vi "MainCode.vi"() -> ()   [LabVIEW 2022 SP3]
uses:
  <vilib>/Instr/_visa.llb/VISA Configure Serial Port (Instr).vi
panel:
  out "Array":string[](array[string])
  in  "Test":bool
  in  "OK Button":bool
  out "read buffer":string="import sensor, image, time\r\n>>> \r\n>>> sensor.reset()\r\n>>> sensor.set_pixformat(sensor.RGB565)\r\nTrue\r\n>>> sensor.set_framesize(sensor.QVGA)  \r\nTrue\r\n>>> sensor.skip_frames(time = 2000)\r\n>>> img = sensor.snapshot()\r\n>>> \r\n>>> \r\n>>> \r\n>>> \r\n>>> "
  out "value":u32[](array[numeric])=[1869639017, 1931506802, 1869835877, 1763716210, 1701273965, 1769218092, 168650093, 540950078, 1044253197, 1702043710, 1919906670, 1936028206, 690517093, 1044253197, 1702043710, 1919906670, 1952805678, 2020175967, 1836216166, 1932031073, 1869835877, 1196568178, 892745026, 1409944873, 224753010, 1044266506, 1852142368, 779251571, 1601463667, 1835102822, 2053731173, 1702045797, 1919906670, 1196839214, 538978625, 1918110221, 168650101, 540950078, 1936614771, 1932423791, 1601202539, 1835102822, 1948808037, 543518057, 808591421, 220803120, 1044266506, 1735223584, 1931492640, 1869835877, 1853042290, 1752395873, 690517103, 1044253197, 168632382, 540950078, 1044253197, 168632382, 540950078, 1044253197] format="%.0x"
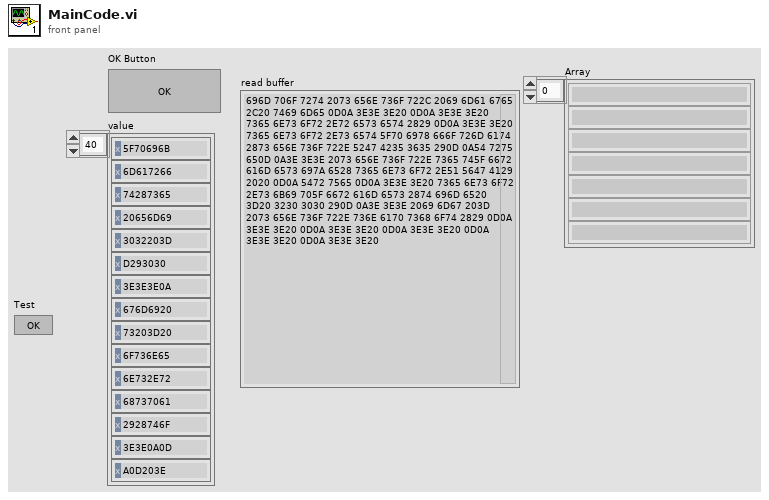
[diagram p1: front panel]
types:
  T1 = enum16{"big-endian, network order", "native, host order", "little-endian"}
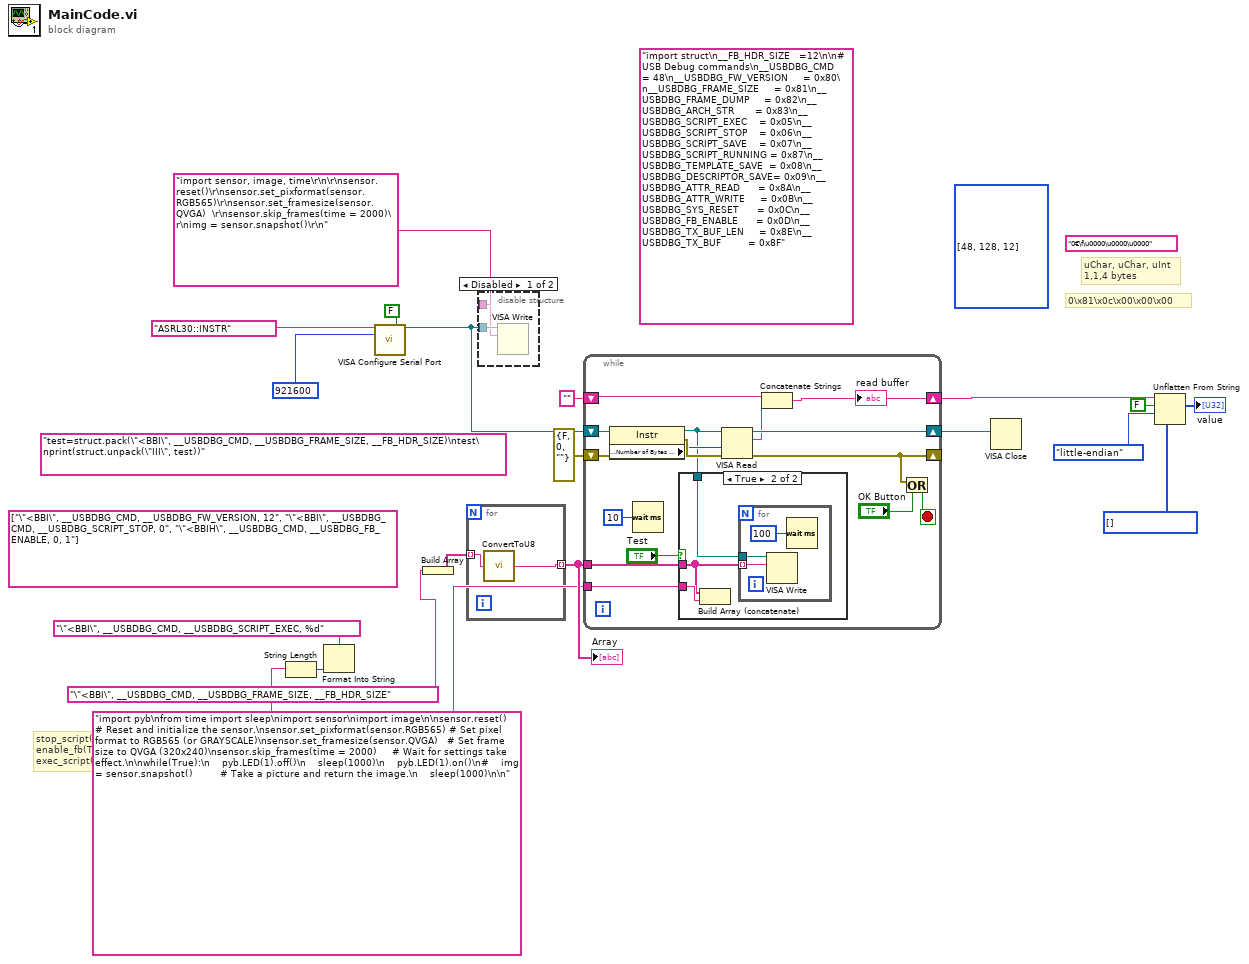
[diagram p0: block diagram]
diagram:
  w3 = "import pyb\nfrom time import sleep\nimport sensor\nimport image\n\nsensor.reset()                      # Reset and initialize the sensor.\nsensor.set_pixformat(sensor.RGB565) # Set pixel format to RGB565 (or GRAYSCALE)\nsensor.set_framesize(sensor.QVGA)   # Set frame size to QVGA (320x240)\nsensor.skip_frames(time = 2000)     # Wait for settings take effect.\n\nwhile(True):\n    pyb.LED(1).off()\n    sleep(1000)\n    pyb.LED(1).on()\n#    img = sensor.snapshot()         # Take a picture and return the image.\n    sleep(1000)\n\n" ("header buffer")
  (unwired) string[] ["\"<BBI\", __USBDBG_CMD, __USBDBG_FW_VERSION, 12", "\"<BBI\", __USBDBG_CMD, __USBDBG_SCRIPT_STOP, 0", "\"<BBIH\", __USBDBG_CMD, __USBDBG_FB_ENABLE, 0, 1"]
  (unwired) i32[] [48, 128, 12]
  (unwired) "0€\f\u0000\u0000\u0000" ("Last")
  (unwired) "test=struct.pack(\"<BBI\", __USBDBG_CMD, __USBDBG_FRAME_SIZE, __FB_HDR_SIZE)\ntest\nprint(struct.unpack(\"III\", test))" ("write buffer")
  (unwired) "import struct\n__FB_HDR_SIZE   =12\n\n# USB Debug commands\n__USBDBG_CMD            = 48\n__USBDBG_FW_VERSION     = 0x80\n__USBDBG_FRAME_SIZE     = 0x81\n__USBDBG_FRAME_DUMP     = 0x82\n__USBDBG_ARCH_STR       = 0x83\n__USBDBG_SCRIPT_EXEC    = 0x05\n__USBDBG_SCRIPT_STOP    = 0x06\n__USBDBG_SCRIPT_SAVE    = 0x07\n__USBDBG_SCRIPT_RUNNING = 0x87\n__USBDBG_TEMPLATE_SAVE  = 0x08\n__USBDBG_DESCRIPTOR_SAVE= 0x09\n__USBDBG_ATTR_READ      = 0x8A\n__USBDBG_ATTR_WRITE     = 0x0B\n__USBDBG_SYS_RESET      = 0x0C\n__USBDBG_FB_ENABLE      = 0x0D\n__USBDBG_TX_BUF_LEN     = 0x8E\n__USBDBG_TX_BUF         = 0x8F" ("write buffer")
  # "\"<BBI\", __USBDBG_CMD, __USBDBG_SCRIPT_EXEC, len(buf))"
  # "stop_script()\nenable_fb(True)\nexec_script(script)"
  # "uChar, uChar, uInt\n1,1,4 bytes"
  # "0\\x81\\x0c\\x00\\x00\\x00"
  n1 = String Length(string=w3) -> (length=w4:i32)
  n2 = Format Into String(format string="\"<BBI\", __USBDBG_CMD, __USBDBG_SCRIPT_EXEC, %d" ("write buffer"), w4) -> ()  [unwired: 2 in, 2 out]
  n3 = call-poly "VISA Configure Serial Port"("VISA resource name"="ASRL30::INSTR" ("Serial Address"), "Enable Termination\nChar (T)"=FALSE ("Enable Termination\nChar (T)"), "baud rate (9600)"=u32 921600 ("baud rate (115200)")) -> ("VISA resource name out"=w12:refnum<visa-resource-name>)  [unwired: 11 in, 1 out]
  n4 = Build Array("\"<BBI\", __USBDBG_CMD, __USBDBG_FRAME_SIZE, __FB_HDR_SIZE" ("write buffer")) -> (w2:string[])
  n5 = for {
    tunnel: [w20] -> w6 mode=indexing
    tunnel: w2 -> [w21] mode=indexing
    n6 = call "ConvertToU8.vi"("struct"=w21) -> ("Binary"=w20:string)
  }
  "Array" <- w6
  n7 = disable-structure shown="Disabled" {
    disable-tunnel: w12 -> [w23 _]
    disable-tunnel: "import sensor, image, time\r\n\r\nsensor.reset()\r\nsensor.set_pixformat(sensor.RGB565)\r\nsensor.set_framesize(sensor.QVGA)  \r\nsensor.skip_frames(time = 2000)\r\nimg = sensor.snapshot()\r\n" ("write buffer") -> [w22 _]
    frame Disabled {
      n8 = VISA Write(VISA resource name=w23, write buffer=w22) -> ()  [unwired: 1 in, 3 out]
    }
    frame Enabled {
    }
  }
  n9 = while {
    shift-right: [w39] -> w10
    shift-left: w12 -> [w38]
    shift-right: [w30] -> _
    shift-left: errorcluster {"status"=FALSE, "code"=0, "source"=""} ("error out") -> [w37]
    shift-right: [w33] -> w8
    shift-left: "" -> [w35]
    tunnel: w6 -> [w26]
    tunnel: w3 -> [w24]
    stop <- w29 stop-if-true
    n10 = property class="Instr"(reference=w38, error in=w37) -> (reference out=w27:refnum<visa-resource-name>, error out=w36:errorcluster, "Serial Settings:Number of Bytes at Serial Port"=w32:u32)
    n11 = Wait (ms)(milliseconds to wait=u32 10) -> ()  [unwired: 1 out]
    n12 = case shown="True" "Test" {
      tunnel: w27 -> [_ w42]
      tunnel: w26 -> [_ w40]
      tunnel: w24 -> [_ w41]
      frame False {
      }
      frame True {
        n13 = Build Array (concatenate)(w40, w41) -> ()  [unwired: 1 out]
        n14 = for {
          tunnel: w42 -> [w45]
          tunnel: w40 -> [w44] mode=indexing
          n15 = VISA Write(VISA resource name=w45, write buffer=w44) -> ()  [unwired: 1 in, 3 out]
          n16 = Wait (ms)(milliseconds to wait=u32 100) -> ()  [unwired: 1 out]
        }
      }
    }
    n17 = VISA Read(VISA resource name=w27, byte count=w32, error in (no error)=w36) -> (VISA resource name out=w39:refnum<visa-resource-name>, read buffer=w34:string, error out=w30:errorcluster)  [unwired: 1 out]
    n18 = Concatenate Strings(w35, w34) -> (w33:string)
    "read buffer" <- w33
    n19 = Or(x=w30, y="OK Button") -> (x .or. y?=w29:bool)
  }
  n20 = VISA Close(VISA resource name=w10) -> ()  [unwired: 1 in, 1 out]
  n21 = Unflatten From String(type=u8[] [], binary string=w8, data includes array or string size? (T)=FALSE, byte order (0:big-endian, network order)=T1."little-endian") -> (value=→"value":u8[])  [unwired: 1 in, 2 out]
